vi "FlatToRichcif_pluginloader_DiscoverResponse.vi"(5 "OutputClusterType":T1, 11 "InputCluster":T6) -> (3 "OutputCluster":T1)   [LabVIEW 2021, in "CIF_PluginLoader_client.lvlib"]
uses:
  CIF_PluginLoader_client.lvlib
  cif_pluginloader_DiscoverResponse_Flat.ctl
  cif_pluginloader_DiscoveredPlugin_Flat.ctl
  cif_common_Version_Flat.ctl
  cif_management_common_PluginMetadata_Flat.ctl
  cif_common_Status_Flat.ctl
  cif_pluginloader_DiscoverResponse.ctl
  cif_pluginloader_DiscoveredPlugin.ctl
  cif_common_Version.ctl
  cif_management_common_PluginMetadata.ctl
  cif_common_Status.ctl
  FlatToRichcif_common_Version.vi
  FlatToRichcif_management_common_PluginMetadata.vi
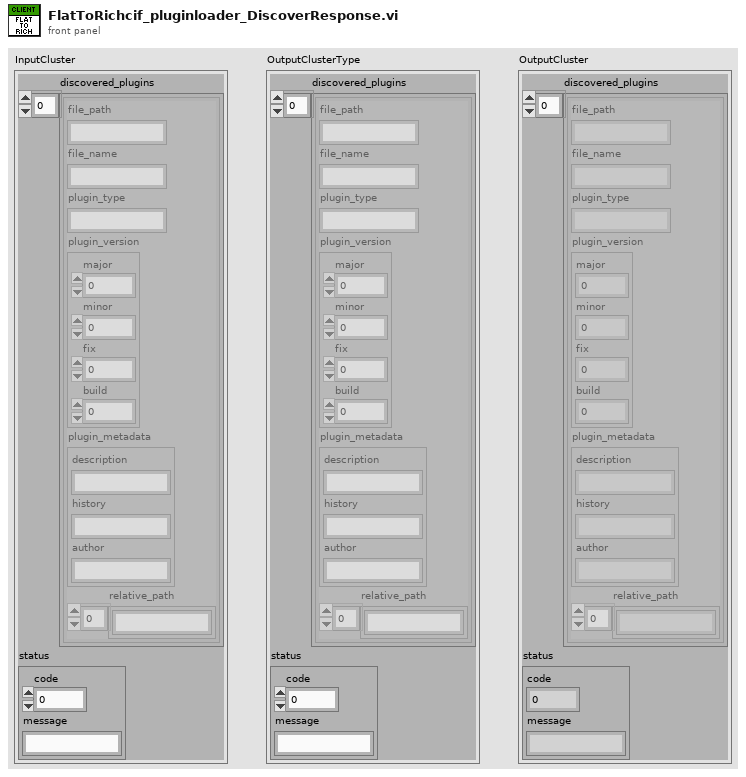
[diagram p1: front panel]
types:
  T1 = typedef "CIF_PluginLoader_client.lvlib/cif_pluginloader_DiscoverResponse.ctl" = cluster{"discovered_plugins":T2[], "status":T5}
  T2 = typedef "CIF_PluginLoader_client.lvlib/cif_pluginloader_DiscoveredPlugin.ctl" = cluster{"file_path":string, "file_name":string, "plugin_type":string, "plugin_version":T3, "plugin_metadata":T4, "relative_path":string[]}
  T3 = typedef "CIF_PluginLoader_client.lvlib/cif_common_Version.ctl" = cluster{"major":u32, "minor":u32, "fix":u32, "build":u32}
  T4 = typedef "CIF_PluginLoader_client.lvlib/cif_management_common_PluginMetadata.ctl" = cluster{"description":string, "history":string, "author":string}
  T5 = typedef "CIF_PluginLoader_client.lvlib/cif_common_Status.ctl" = cluster{"code":i32, "message":string}
  T6 = typedef "CIF_PluginLoader_client.lvlib/cif_pluginloader_DiscoverResponse_Flat.ctl" = cluster{"discovered_plugins":T7[], "status":T10}
  T7 = typedef "CIF_PluginLoader_client.lvlib/cif_pluginloader_DiscoveredPlugin_Flat.ctl" = cluster{"file_path":string, "file_name":string, "plugin_type":string, "plugin_version":T8, "plugin_metadata":T9, "relative_path":string[]}
  T8 = typedef "CIF_PluginLoader_client.lvlib/cif_common_Version_Flat.ctl" = cluster{"major":u32, "minor":u32, "fix":u32, "build":u32}
  T9 = typedef "CIF_PluginLoader_client.lvlib/cif_management_common_PluginMetadata_Flat.ctl" = cluster{"description":string, "history":string, "author":string}
  T10 = typedef "CIF_PluginLoader_client.lvlib/cif_common_Status_Flat.ctl" = cluster{"code":i32, "message":string}
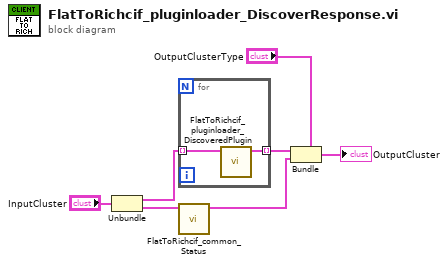
[diagram p0: block diagram]
diagram:
  n1 = Unbundle "Unbundle"("InputCluster") -> ("discovered_plugins"=w4:T7[], "status"=w2:T10)
  n2 = for {
    tunnel: w4 -> [w9] mode=indexing
    tunnel: [w8] -> w3 mode=indexing
    n3 = call "FlatToRichcif_pluginloader_DiscoveredPlugin.vi"("InputCluster"=w9) -> ("OutputCluster"=w8:T2)  [unwired: 10 in]
  }
  n4 = call "FlatToRichcif_common_Status.vi"("InputCluster"=w2) -> ("OutputCluster"=w1:T5)  [unwired: 10 in]
  n5 = Bundle "Bundle"(cluster="OutputClusterType", "discovered_plugins"=w3, "status"=w1) -> (→"OutputCluster":T1)
